vi "Get_Instrument_Class.vi"(8 "error in":errorcluster, 11 "Instrument_ID":string) -> (0 "error out":errorcluster, 3 "Instrument class path":path)   [LabVIEW 2020, in "Pin_Instrument_Factory.lvclass"]
uses:
  Pin_Instrument_Factory.lvclass
  <vilib>/Utility/config.llb/Read Key (String).vi
  <vilib>/Utility/config.llb/NI_LVConfig.lvlib
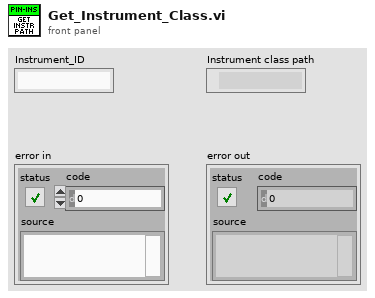
[diagram p1: front panel]
types:
  T1 = typedef "Pin_Instrument_Factory.lvclass/Paths.ctl" = cluster{"Instr_Class_Mapping":path, "Instr_Class_base_path":path}
  T2 = typedef "NI_LVConfig.lvlib/Config Data RefNum.ctl" = refnum<k1>
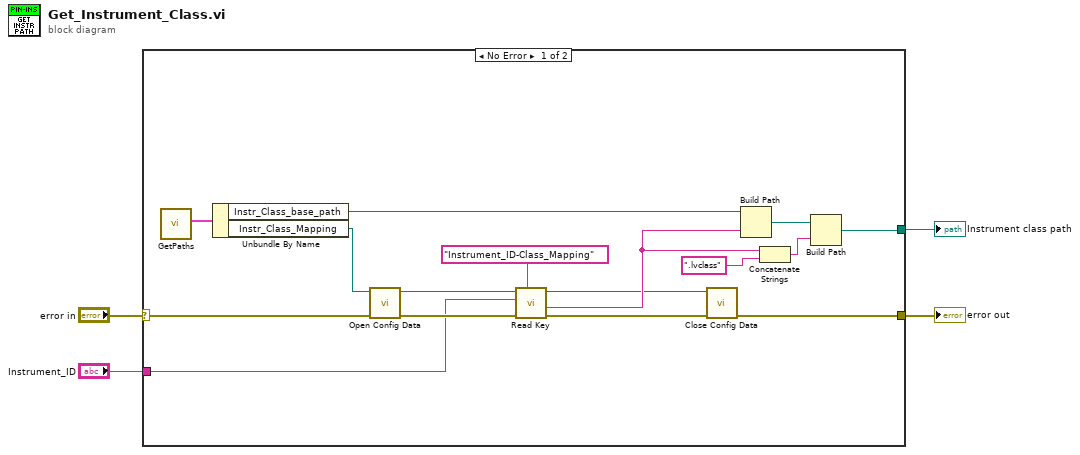
[diagram p0: block diagram]
diagram:
  n1 = case shown="No Error" "error in" {
    selector: "error in" -> [w20 w21]
    tunnel: [w6 w21] -> w3
    tunnel: "Instrument_ID" -> [w14 _]
    tunnel: [w7 _] -> w1
    frame No Error {
      n2 = call "GetPaths.vi"() -> ("Paths"=w18:T1)  [unwired: 11 in]
      n3 = Unbundle By Name(w18) -> ("Instr_Class_base_path"=w12:path, "Instr_Class_Mapping"=w17:path)
      n4 = call <vilib>:"Open Config Data.vi"("error in (no error)"=w20, "configuration file path"=w17) -> ("error out"=w19:errorcluster, "refnum"=w15:T2)  [unwired: 7 in, 1 out]
      n5 = call-poly <vilib>:"Read Key.vi"("section"="Instrument_ID-Class_Mapping", "error in (no error)"=w19, "key"=w14, "refnum"=w15) -> ("error out"=w16:errorcluster, "value"=w9:string, "refnum out"=w5:T2)  [unwired: 4 in, 1 out]
      n6 = call <vilib>:"Close Config Data.vi"("error in (no error)"=w16, "refnum"=w5) -> ("error out"=w6:errorcluster)  [unwired: 8 in, 1 out]
      n7 = Build Path(base path=w12, name or relative path=w9) -> (appended path=w11:path)
      n8 = Concatenate Strings(w9, ".lvclass" ("string")) -> (w8:string)
      n9 = Build Path(base path=w11, name or relative path=w8) -> (appended path=w7:path)
    }
    frame Error {
    }
  }
  "error out" <- w3
  "Instrument class path" <- w1
